vi "Read TcpClient.vi"(8 "error in (no error)":errorcluster, 11 "dotNET TCP Socket in":refnum<class "dotNET TCP Socket.lvclass">) -> (0 "error out":errorcluster, 2 "TcpClient":refnum<k24>, 3 "dotNET TCP Socket out":refnum<class "dotNET TCP Socket.lvclass">)   [LabVIEW 2013, in "dotNET SSL Socket.lvlib" / "dotNET TCP Socket.lvclass"]
uses:
  dotNET TCP Socket.lvclass
  dotNET TCP Socket.lvclass/dotNET TCP Socket.ctl
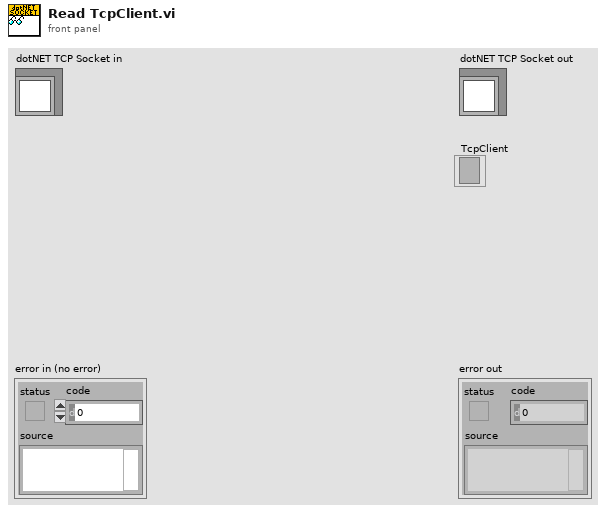
[diagram p1: front panel]
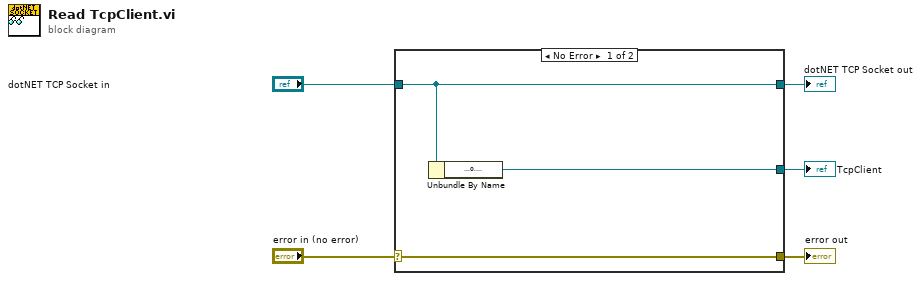
[diagram p0: block diagram]
diagram:
  n1 = case shown="No Error" "error in (no error)" {
    selector: "error in (no error)" -> [w8 w9]
    tunnel: [w8 w9] -> w4
    tunnel: [w7 w10] -> w2
    tunnel: "dotNET TCP Socket in" -> [w7 w10]
    tunnel: [w6 _] -> w1
    frame No Error {
      n2 = Unbundle By Name(w7) -> ("TcpClient"=w6:refnum<k24>)
    }
    frame Error {
    }
  }
  "error out" <- w4
  "dotNET TCP Socket out" <- w2
  "TcpClient" <- w1
